vi "Configure test.vi"(6 "Assert VI Path":path, 7 "Existing Queue Elements":string, 8 "error in (no error)":errorcluster, 11 "Basic Int GT in":refnum<class "Int GT.lvclass">) -> (0 "error out":errorcluster, 3 "Basic Int GT out":refnum<class "Int GT.lvclass">)   [LabVIEW 2018, in "Int GT.lvclass"]
uses:
  Int GT.lvclass
  360f313f-2adf-4ed9-8ff9-9f793de8b156.vi
  <vilib>/JDP Science/JSONtext/Find Item.vi
  360f313f-2adf-4ed9-8ff9-9f793de8b156.vi/ab53348d-bf09-4c02-b8f0-70f3e4ef24c9.vi
  360f313f-2adf-4ed9-8ff9-9f793de8b156.vi/f947ec25-d6ae-4896-95dd-cb9cf55c942e.vi
  <vilib>/JDP Science/JSONtext/String Subset.vi
  Test Class String IDs.vi
  <vilib>/JDP Science/JSONtext/Parsing/Parse Full Path or Item Name.vi
  <vilib>/JDP Science/JSONtext/Offset/Find Item Locations by Path.vi
  <vilib>/JDP Science/JSONtext/JSON text to Variant.vi
  <vilib>/JDP Science/JSONtext/Variant to JSON Text.vi
  <vilib>/JDP Science/JSONtext/Set Item.vi
  Integer.lvclass
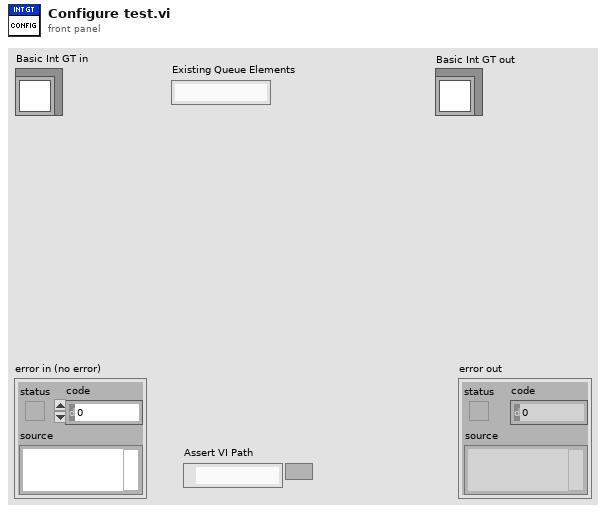
[diagram p1: front panel]
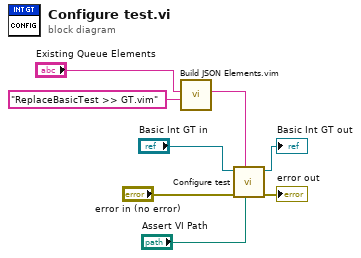
[diagram p0: block diagram]
diagram:
  n1 = call "Build JSON Elements.vim"("Append Element(s)"="ReplaceBasicTest >> GT.vim", "JSON Elements in ({})"="Existing Queue Elements") -> ("JSON Elements out"=w1:string)  [unwired: 9 in]
  n2 = call-parent "Configure test.vi"("Assert VI Path"="Assert VI Path", "Existing Queue Elements"=w1, "error in (no error)"="error in (no error)", "Basic Integer in"="Basic Int GT in") -> ("error out"=→"error out":errorcluster, "Basic Integer out"=→"Basic Int GT out":refnum<class "Int GT.lvclass">)  [unwired: 6 in]
